vi "GetShotNumber(viaTreeString).vi"(1 "Tree Name":string) -> (0 "Shot #":string)   [LabVIEW 2013]
uses:
  <vilib>/MDSplus/Classes/Tree_Class/Tree.lvclass
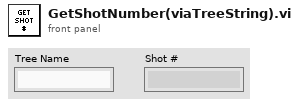
[diagram p1: front panel]
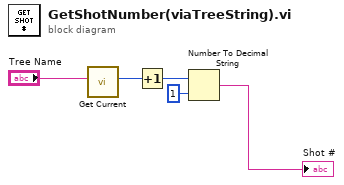
[diagram p0: block diagram]
diagram:
  n1 = call <vilib>:"Get Current.vi"("Tree name"="Tree Name") -> ("Current shot out"=w4:i32)  [unwired: 8 in, 2 out]
  n2 = Increment(x=w4) -> (x+1=w5:i32)
  n3 = Number To Decimal String(number=w5, width (-)=i16 1) -> (decimal integer string=→"Shot #":string)
